vi "Configure BERT.vi"(6 "Total Bits (10000)":u32=10000, 7 "Stop Threshold (100)":u32=100, 8 "error in (no error)":errorcluster, 9 "Stop Threshold Criteria (1: None)":i32(ring)=1 items=["Bit Errors", "None"], 10 "Enable BERT (F: Disable)":bool, 11 "VISA resource name":refnum<visa-resource-name>) -> (0 "error out":errorcluster, 3 "VISA resource name out":refnum<visa-resource-name>)   [LabVIEW 2018, in "Agilent PSG MXG Series.lvlib"]
doc: "Configures the bit error rate test state, stop threshold and total bits in one measurement.\n\n<b>Note:</b>\nIt is applicable for N5172B/82B with <b>Option UN7</b> only."
uses:
  Agilent PSG MXG Series.lvlib
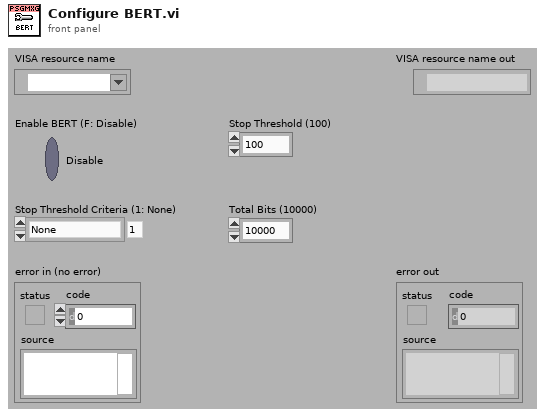
[diagram p1: front panel]
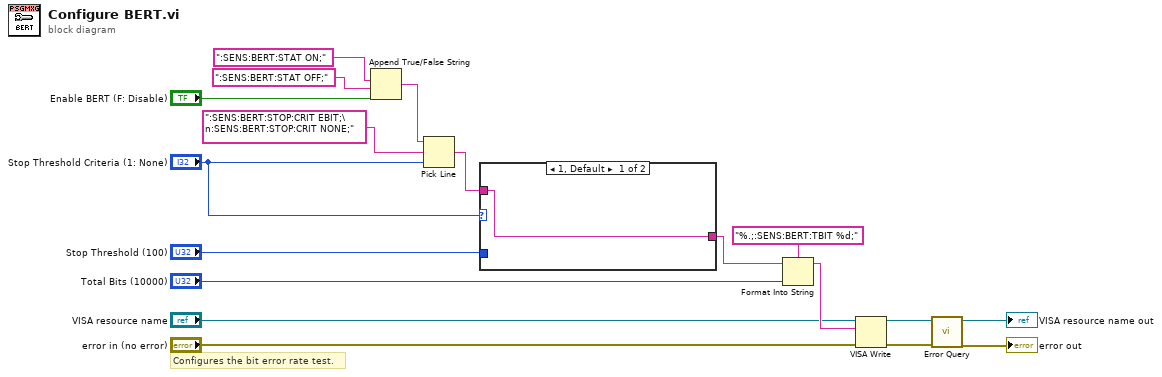
[diagram p0: block diagram]
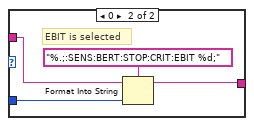
[diagram p2: hidden frame]
diagram:
  # "Configures the bit error rate test."
  n1 = Append True/False String(1:"Enable BERT (F: Disable)", 2:":SENS:BERT:STAT OFF;", 3:":SENS:BERT:STAT ON;") -> (0:w14:string)  [unwired: 1 in]
  n2 = Pick Line(string ("")=w14, multi-line string=":SENS:BERT:STOP:CRIT EBIT;\n:SENS:BERT:STOP:CRIT NONE;", line index="Stop Threshold Criteria (1: None)") -> (output string=w13:string)
  n3 = case shown="1, Default" "Stop Threshold Criteria (1: None)" {
    tunnel: w13 -> [w19 w23]
    tunnel: "Stop Threshold (100)" -> [_ w21]
    tunnel: [w19 w20] -> w11
    frame 1, Default {
    }
    frame 0 {
      # "EBIT is selected"
      n4 = Format Into String(format string="%.;:SENS:BERT:STOP:CRIT:EBIT %d;", initial string=w23, w21) -> (resulting string=w20:string)  [unwired: 1 in, 1 out]
    }
  }
  n5 = Format Into String(format string="%.;:SENS:BERT:TBIT %d;", initial string=w11, "Total Bits (10000)") -> (resulting string=w8:string)  [unwired: 1 in, 1 out]
  n6 = VISA Write(VISA resource name="VISA resource name", write buffer=w8, error in (no error)="error in (no error)") -> (VISA resource name out=w5:refnum<visa-resource-name>, error out=w4:errorcluster)  [unwired: 1 out]
  n7 = call "Error Query.vi"("error in (no error)"=w4, "VISA resource name"=w5) -> ("error out"=→"error out":errorcluster, "VISA resource name out"=→"VISA resource name out":refnum<visa-resource-name>)  [unwired: 6 in, 2 out]
